vi "Switch_CheckConnect.vi"(10 "COM":refnum<visa-resource-name> caption="VISA资源名称") -> (2 "通信成功？":bool)   [LabVIEW 2018, in "Switch.lvlib"]
uses:
  Switch.lvlib
panel:
  # "看能否接收到一帧数据"
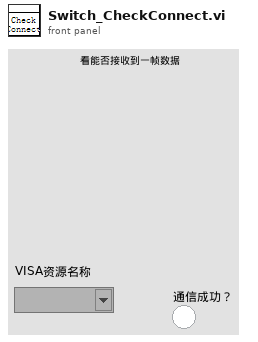
[diagram p1: front panel]
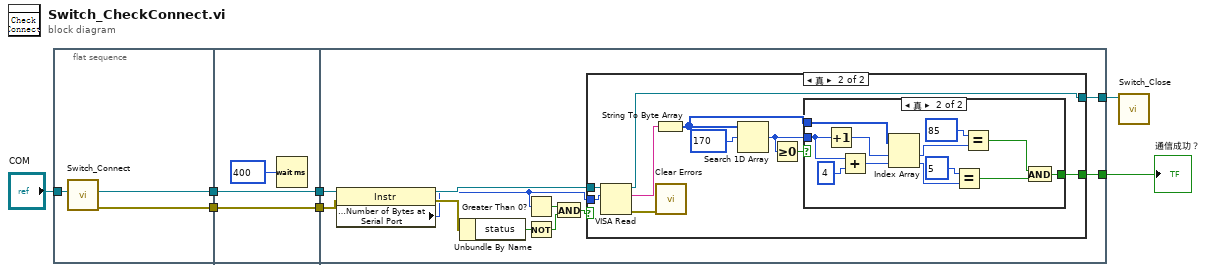
[diagram p0: block diagram]
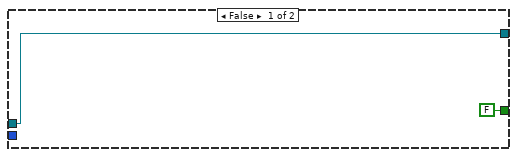
[diagram p2: hidden frame]
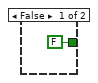
[diagram p3: hidden frame]
diagram:
  n1 = flat-sequence {
    tunnel: "COM" -> [w10]
    tunnel: [w9] -> w5
    tunnel: [w8] -> w3
    tunnel: [w12] -> w6
    tunnel: w5 -> [w12]
    tunnel: [w11] -> w4
    tunnel: w3 -> [w11]
    tunnel: w6 -> [w23]
    tunnel: w4 -> [w22]
    tunnel: [w16] -> w2
    tunnel: [w15] -> w1
    frame #0 {
      n2 = call "Switch_Connect.vi"("COM"=w10) -> ("error out"=w8:errorcluster, "COM Out"=w9:refnum<visa-resource-name>)  [unwired: 9 in]
    }
    frame #1 {
      n3 = Wait (ms)(milliseconds to wait=u32 400 ("等待时间（毫秒）")) -> ()  [unwired: 1 out]
    }
    frame #2 {
      n4 = property class="Instr"(reference=w23, error in=w22) -> (reference out=w24:refnum<visa-resource-name>, error out=w19:errorcluster, "Serial Settings:Number of Bytes at Serial Port"=w14:u32)
      n5 = Unbundle By Name(w19) -> ("status"=w18:bool)
      n6 = Greater Than 0?(x=w14) -> (x > 0?=w21:bool)
      n7 = Not(x=w18) -> (.not. x?=w17:bool)
      n8 = And(x=w21, y=w17) -> (x .and. y?=w20:bool)
      n9 = case shown="真" w20 {
        tunnel: w24 -> [w25 w34]
        tunnel: [FALSE w32] -> w16
        tunnel: [w25 w31] -> w15
        tunnel: w14 -> [_ w28]
        frame False {
        }
        frame True {
          n10 = VISA Read(VISA resource name=w34, byte count=w28) -> (VISA resource name out=w31:refnum<visa-resource-name>, read buffer=w36:string, error out=w27:errorcluster)  [unwired: 1 in, 1 out]
          n11 = String To Byte Array(string=w36) -> (unsigned byte array=w29:u8[])
          n12 = call <vilib>:"Clear Errors.vi"("error in (no error)"=w27) -> ()  [unwired: 5 in, 2 out]
          n13 = Search 1D Array(1D array=w29, element=u8 170 ("元素")) -> (index of element=w30:i32)  [unwired: 1 in]
          n14 = Greater Or Equal To 0?(x=w30) -> (x >= 0?=w33:bool)
          n15 = case shown="真" w33 {
            tunnel: [FALSE w42] -> w32
            tunnel: w30 -> [_ w38]
            tunnel: w29 -> [_ w40]
            frame False {
            }
            frame True {
              n16 = Increment(x=w38) -> (x+1=w48:i32)
              n17 = Add(x=w38, y=4) -> (x+y=w46:i32)
              n18 = Index Array(array=w40, index #1=w48, index #2=w46) -> (element #1=w41:u8, element #2=w39:u8)
              n19 = Equal?(x=u8 5 ("元素"), y=w39) -> (x = y?=w44:bool)
              n20 = Equal?(x=u8 85 ("元素"), y=w41) -> (x = y?=w43:bool)
              n21 = And(x=w43, y=w44) -> (x .and. y?=w42:bool)
            }
          }
        }
      }
    }
  }
  n22 = call "Switch_Close.vi"("COM"=w1) -> ()  [unwired: 10 in, 1 out]
  "通信成功？" <- w2
